vi "Event Identifier.vi"(8 "error in (no error)":errorcluster, 11 "Example Custom ID in":refnum<class "Example Custom ID.lvclass">) -> (0 "error out":errorcluster, 2 "Event Identifier":string)   [LabVIEW 2020, in "serenial.io-ase.example.lvlib" / "Example Custom ID.lvclass"]
uses:
  Example Custom ID.lvclass
  Example Custom ID.lvclass/Example Custom ID.ctl
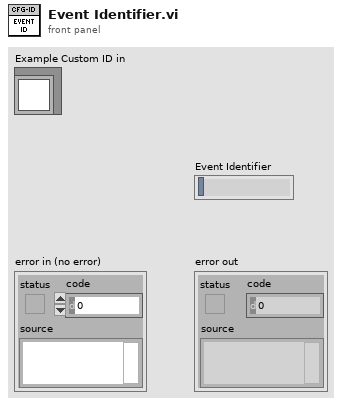
[diagram p1: front panel]
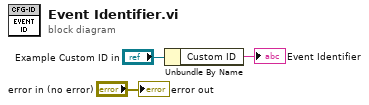
[diagram p0: block diagram]
diagram:
  n1 = Unbundle By Name("Example Custom ID in") -> ("Custom ID"=→"Event Identifier":string)
  "error out" <- "error in (no error)"
